vi "Z_Scan_v12 (SubVI).vi"(0 "Scan Axis":string, 1 "Scan Termination":T1(ring), 2 "Center of Scan":bool, 3 "Scan Type":enum16{"Sinusoidal", "Spiral"}(ring), 4 "Analog Input":i32, 5 "Table rate":i32, 6 "System no.":i32, 7 "error in (no error)":errorcluster, 8 "Z Mesh":dbl, 9 "Z-frequency":dbl, 10 "X Scan Range":dbl, 11 "Z-velocity":dbl, 12 "Z Scan Range":dbl, 14 "X Scan Center":dbl, 16 "Z Scan Center":dbl) -> (18 "3D Line Graph":refnum<class "Base Datatype.lvclass">[](array[class]), 20 "Intensity Graph":dbl[][](array[numeric]), 25 "Nano AS Data":dbl[][](array[numeric]), 26 "AS Duration (msec)":u32, 27 "error out":errorcluster)   [LabVIEW 2023]
uses:
  <vilib>/Native 3D Graph/classes/Base Datatype.lvclass
  <vilib>/Native 3D Graph/xcontrol/3DPC_SurfacePlot.xctl
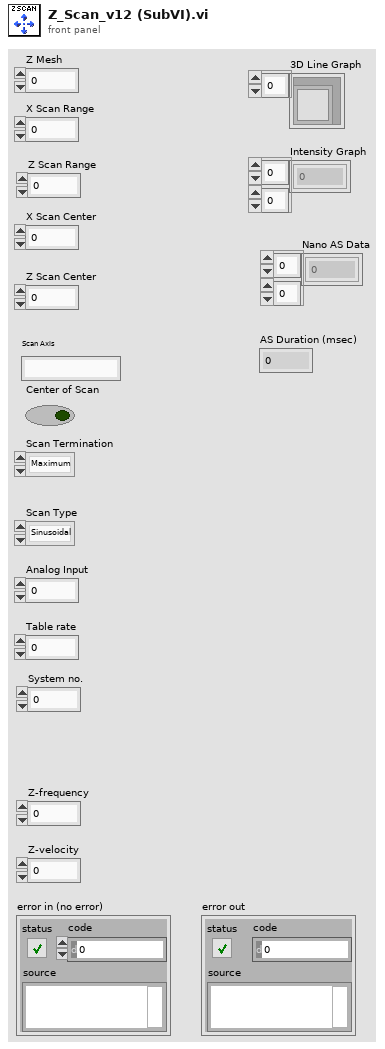
[diagram p1: front panel]
types:
  T1 = enum16{"Maximum", "End Position", "Center of scan", ""}
  T2 = cluster{"Set target type?":bool, "Target type":i32}
  T3 = cluster{"Set stop pos. option?":bool, "Stop pos. option":i32}
  T4 = cluster{"Set centroid method?":bool, "Centroid method":i32}
  T5 = cluster{"Step axis":string, "Range step axis":dbl, "Set Mid. pos?":bool, "Mid. pos. step axis":dbl}
  T6 = cluster{"Scan axis":string, "Range scan axis":dbl, "Set Mid. pos?":bool, "Mid. pos. scan axis":dbl}
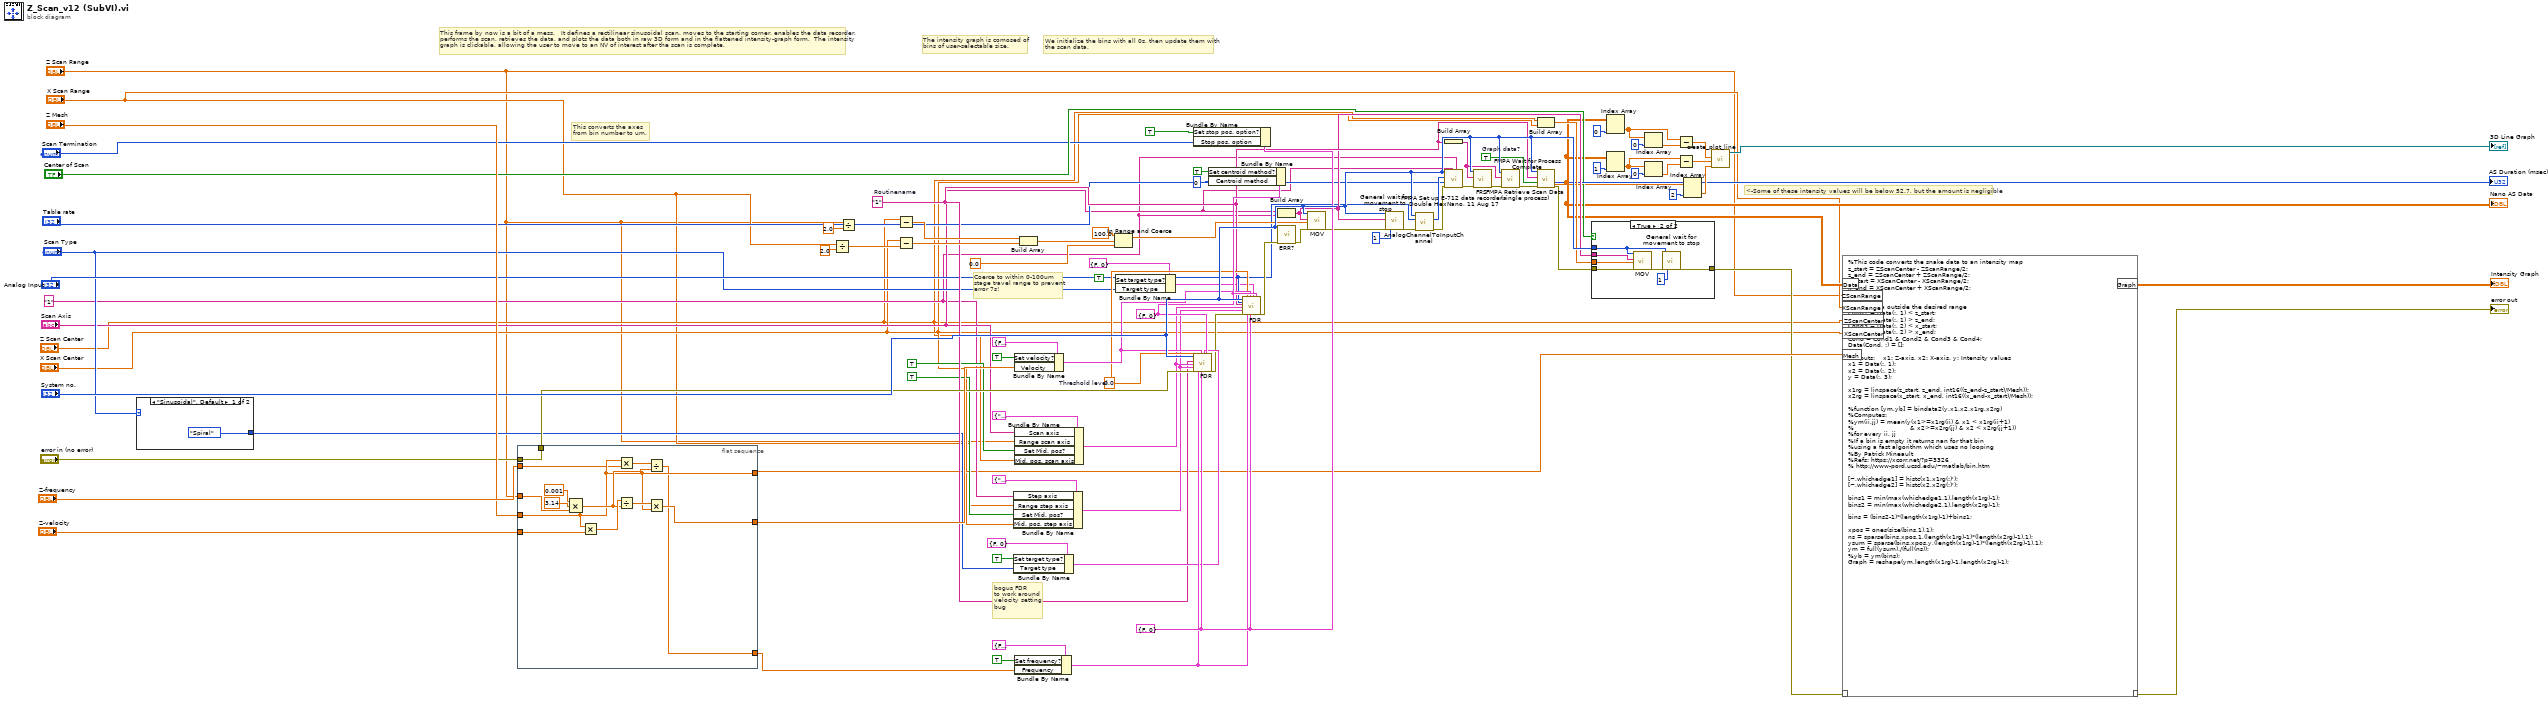
[diagram p0: block diagram]
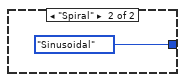
[diagram p2: hidden frame]
diagram:
  w11 = "1"
  w44 = TRUE  # Graph data?
  w76 = T3 {"Set stop pos. option?"=FALSE, "Stop pos. option"=0} ("Stop position option settings")
  w74 = T4 {"Set centroid method?"=FALSE, "Centroid method"=0} ("Centroid method settings")
  w72 = 0.0  # Threshold level
  w66 = "1"  # Routinename
  # "<-Some of these intensity values will be below 52.7, but the amount is negligible"
  # "This converts the axes\nfrom bin number to um."
  # "We initialize the bins with all 0s, then update them with\nthe scan data."
  # "The intensity graph is comosed of\nbins of user-selectable size."
  # "This frame by now is a bit of a mess.   It defines a rectilinear sinusoidal scan, moves to the starting corner, enables the data recorder,\nperforms the scan, retrieves the data, and plots the data both in raw 3D form and in the flattened intensity-graph form.  The intensity\ngraph is clickable, allowing the user to move to an NV of interest after the scan is complete."
  # "bogus FDR\nto work around\nvelocity setting\nbug"
  # "Coerce to within 0-100um\nstage travel range to prevent\nerror 7s!"
  n1 = case shown="\"Sinusoidal\", Default" "Scan Type" {
    tunnel: [enum16{"Sinusoidal", "Spiral"}."Spiral" ("Scan Type") enum16{"Sinusoidal", "Spiral"}."Sinusoidal" ("Scan Type")] -> w16
    frame "Sinusoidal", Default {
    }
    frame "Spiral" {
    }
  }
  n2 = flat-sequence {
    tunnel: "Z Scan Range" -> [w102]
    tunnel: [w98] -> w82
    tunnel: "error in (no error)" -> [w98]
    tunnel: "Z Mesh" -> [w97]
    tunnel: "Z-frequency" -> [w96]
    tunnel: "Z-velocity" -> [w95]
    tunnel: [w97] -> w9
    tunnel: [w94] -> w90
    tunnel: [w93] -> w89
    frame #0 {
      n3 = Compound Arithmetic op=MULTIPLY(0.001, 3.14, w102) -> (w100:dbl)
      n4 = Multiply(x=w97, y=w95) -> (x*y=w101:dbl)
      n5 = Multiply(x=w97, y=w96) -> (x*y=w105:dbl)
      n6 = Divide(x=w101, y=w100) -> (x/y=w99:dbl)
      n7 = Divide(x=w105, y=w100) -> (x/y=w93:dbl)
      n8 = Multiply(x=w99, y=w97) -> (x*y=w94:dbl)
    }
  }
  n9 = Divide(x="X Scan Range", y=2.0) -> (x/y=w64:dbl)
  n10 = Divide(x="Z Scan Range", y=2.0) -> (x/y=w32:dbl)
  n11 = Subtract(x="Z Scan Center", y=w32) -> (x-y=w85:dbl)
  n12 = Subtract(x="X Scan Center", y=w64) -> (x-y=w86:dbl)
  n13 = Bundle By Name(cluster=T5 {"Step axis"="", "Range step axis"=0.1, "Set Mid. pos?"=FALSE, "Mid. pos. step axis"=0.1} ("Step axis settings"), "Step axis"=w11, "Range step axis"="X Scan Range", "Set Mid. pos?"=TRUE, "Mid. pos. step axis"="X Scan Center") -> (w67:T5)
  n14 = Bundle By Name(cluster=T2 {"Set target type?"=FALSE, "Target type"=0} ("Target type settings"), "Set target type?"=TRUE, "Target type"=w16) -> (w71:T2)
  n15 = Bundle By Name(cluster=cluster{"Set velocity?":bool, "Velocity":dbl} {"Set velocity?"=FALSE, "Velocity"=0.1} ("Velocity settings"), "Set velocity?"=TRUE ("Set target type?"), "Velocity"=w90) -> (w73:cluster{"Set velocity?":bool, "Velocity":dbl})
  n16 = Bundle By Name(cluster=T6 {"Scan axis"="", "Range scan axis"=0.1, "Set Mid. pos?"=FALSE, "Mid. pos. scan axis"=0.1} ("Scan axis settings"), "Scan axis"="Scan Axis", "Range scan axis"="Z Scan Range", "Set Mid. pos?"=TRUE, "Mid. pos. scan axis"="Z Scan Center") -> (w68:T6)
  n17 = Bundle By Name(cluster=cluster{"Set frequency?":bool, "Frequency":dbl} {"Set frequency?"=FALSE, "Frequency"=10.0} ("Frequency settings"), "Set frequency?"=TRUE, "Frequency"=w89) -> (w75:cluster{"Set frequency?":bool, "Frequency":dbl})
  n18 = Build Array(w85, w86) -> (w62:dbl[])
  n19 = In Range and Coerce(upper limit=100.0, x=w62, lower limit=0.0) -> (coerced(x)=w63:dbl[])  [unwired: 1 out]
  n20 = Bundle By Name(cluster=T2 {"Set target type?"=FALSE, "Target type"=0} ("Target type settings"), "Set target type?"=TRUE, "Target type"="Scan Type") -> (w23:T2)
  n21 = Bundle By Name(cluster=w76, "Set stop pos. option?"=TRUE, "Stop pos. option"="Scan Termination") -> ()  [unwired: 1 out]
  n22 = call "FDR.vi"("System no."="System no.", "Routinename"=w66, "Scan axis settings"=w68, "Step axis settings"=w67, "error in"=w82, "Threshold level"=w72, "Frequency settings"=w75, "Velocity settings"=w73, "Stop position option settings"=w76, "Target type settings"=w71, "Centroid method settings"=w74) -> ("error out"=w65:errorcluster)  [unwired: 3 in, 5 out]
  n23 = Bundle By Name(cluster=w74, "Set centroid method?"=TRUE, "Centroid method"=0) -> ()  [unwired: 1 out]
  n24 = call "FDR.vi"("System no."="System no.", "Board"="Analog Input", "Routinename"=w66, "Scan axis settings"=w68, "Step axis settings"=w67, "error in"=w65, "Threshold level"=w72, "Frequency settings"=w75, "Velocity settings"=w73, "Stop position option settings"=w76, "Target type settings"=w23, "Centroid method settings"=w74) -> ("error out"=w49:errorcluster)  [unwired: 2 in, 5 out]
  n25 = Build Array("Scan Axis", w11) -> (w47:string[])
  n26 = call "ERR?.vi"("System no."="System no.", "error in"=w49) -> ("error out"=w50:errorcluster)  [unwired: 16 in, 1 out]
  n27 = call "MOV.vi"("System no."="System no.", "Axes to move"=w47, "Position values"=w63, "error in"=w50) -> ("error out"=w34:errorcluster)  [unwired: 1 in, 14 out]
  n28 = call "General wait for movement to stop.vi"("System no."="System no.", "Axes to wait for"=w47, "error in"=w34, "Polling cycle \ntime, ms"=u32 1 ("Polling cycle \ntime, ms")) -> ("error out"=w35:errorcluster)  [unwired: 4 in, 11 out]
  n29 = call "AnalogChannelToInputChannel.vi"("error in (no error)"=w35, "Optical Channel In"="Analog Input", "System no."="System no.") -> ("error out"=w38:errorcluster, "Input Channel Out"=w45:i32)  [unwired: 7 in]
  n30 = Build Array(w66) -> (w43:string[])
  n31 = call "FMPA Set up E-712 data recorder - Double HexNano, 11 Aug 17.vi"("Step axis sensor ch"=w11, "Scan axis sensor ch"="Scan Axis", "error in"=w38, "Table rate"="Table rate", "Opt. Ch."=w45, "System no."="System no.") -> ("error out"=w40:errorcluster)  [unwired: 5 in]
  n32 = call "FRS.vi"("System no."="System no.", "Routines to start"=w43, "error in"=w40) -> ("error out"=w41:errorcluster)  [unwired: 16 in]
  n33 = call "FMPA Wait for Process Complete.vi"("error in"=w41, "Routines to query"=w43, "System no."="System no.") -> ("error out"=w42:errorcluster)  [unwired: 7 in, 1 out]
  n34 = Build Array("Z Scan Center", "X Scan Center") -> (w46:dbl[])
  n35 = call "FMPA Retrieve Scan Data (single process).vi"("System no."="System no.", "Process"=w66, "Graph data?"=w44, "error in"=w42) -> ("Duration (msec)"=→"AS Duration (msec)":u32, "Data"=w8:dbl[][], "error out"=w10:errorcluster)  [unwired: 10 in, 3 out]
  "Nano AS Data" <- w8
  n36 = case shown="True" "Center of Scan" {
    tunnel: w46 -> [_ w111]
    tunnel: w47 -> [_ w110]
    tunnel: w10 -> [w106 w109]
    tunnel: "System no." -> [_ w108]
    tunnel: [w106 w107] -> w7
    frame False {
    }
    frame True {
      n37 = call "MOV.vi"("System no."=w108, "Axes to move"=w110, "Position values"=w111, "error in"=w109) -> ("error out"=w113:errorcluster)  [unwired: 1 in, 14 out]
      n38 = call "General wait for movement to stop.vi"("System no."=w108, "error in"=w113, "Polling cycle \ntime, ms"=u32 1 ("Polling cycle \ntime, ms")) -> ("error out"=w107:errorcluster)  [unwired: 5 in, 11 out]
    }
  }
  n39 = Index Array(array=w8, index (col)=0 ("index")) -> (element=w54:dbl[])  [unwired: 1 in]
  n40 = Index Array(array=w8, index (col)=1 ("index")) -> (element=w51:dbl[])  [unwired: 1 in]
  n41 = Index Array(array=w54, index=0) -> (element=w55:dbl)
  n42 = Index Array(array=w51, index=0) -> (element=w52:dbl)
  n43 = Subtract(x=w54, y=w55) -> (x-y=w78:dbl[])
  n44 = Subtract(x=w51, y=w52) -> (x-y=w79:dbl[])
  n45 = Index Array(array=w8, index (col)=2 ("index")) -> (element=w80:dbl[])  [unwired: 1 in]
  n46 = call <vilib>:"create_plot_line.vi"("z vector"=w80, "y vector"=w79, "x vector"=w78) -> ("plots out"=→"3D Line Graph":refnum<class "Base Datatype.lvclass">[])  [unwired: 2 in, 6 out]
  n47 = script code="%This code converts the snake data to an intensity map\nz_start = ZScanCenter - ZScanRange/2;\nz_end = ZScanCenter + ZScanRange/2;\nx_start = XScanCenter - XScanRange/2;\nx_end = XScanCenter + XScanRange/2;\n\n\n%Filter data outside the desired range\nCond1 = Data(:, 1) < z_start;\nCond2 = Data(:, 1) > z_end;\nCond3 = Data(:, 2) < x_start;\nCond4 = Data(:, 2) > x_end;\nCond = Cond1 & Cond2 & Cond3 & Cond4;\nData(Cond, :) = [];\n\n%Inputs:    x1: Z-axis, x2: X-axis, y: Intensity values\nx1 = Data(:, 1);\nx2 = Data(:, 2);\ny = Data(:, 3);\n\nx1rg = linspace(z_start, z_end, int16((z_end-z_start)/Mesh));\nx2rg = linspace(x_start, x_end, int16((x_end-x_start)/Mesh));\n\n%function [ym,yb] = bindata2(y,x1,x2,x1rg,x2rg)\n%Computes:\n%ym(ii,jj) = mean(y(x1>=x1rg(ii) & x1 < x1rg(ii+1) \n%                            & x2>=x2rg(jj) & x2 < x2rg(jj+1))\n%for every ii, jj\n%If a bin is empty it returns nan for that bin\n%using a fast algorithm which uses no looping\n%By Patrick Mineault\n%Refs: https://xcorr.net/?p=3326\n% http://www-pord.ucsd.edu/~matlab/bin.htm\n\n[~,whichedge1] = histc(x1,x1rg(:)');\n[~,whichedge2] = histc(x2,x2rg(:)');\n\nbins1 = min(max(whichedge1,1),length(x1rg)-1);\nbins2 = min(max(whichedge2,1),length(x2rg)-1);\n\nbins = (bins2-1)*(length(x1rg)-1)+bins1;\n\nxpos = ones(size(bins,1),1);\nns = sparse(bins,xpos,1,(length(x1rg)-1)*(length(x2rg)-1),1);\nysum = sparse(bins,xpos,y,(length(x1rg)-1)*(length(x2rg)-1),1);\nym = full(ysum)./(full(ns));\n%yb = ym(bins);\nGraph = reshape(ym,length(x1rg)-1,length(x2rg)-1);"("??"=w7, "Data"=w8, "Mesh"=w9, "ZScanRange"="Z Scan Range", "XScanRange"="X Scan Range", "ZScanCenter"="Z Scan Center", "XScanCenter"="X Scan Center") -> ("??"=→"error out":errorcluster, "Graph"=→"Intensity Graph":dbl[][])
